vi "TextLog-Logging Thread.vi"(7 "length":i32=100000) -> ()   [LabVIEW 2020]
uses:
  TextLog-Queue Data.ctl
  TextLog-Command.ctl
  TextLog-State.ctl
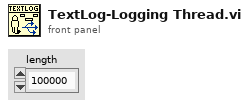
[diagram p1: front panel]
types:
  T1 = typedef "TextLog-State.ctl" = cluster{"path":path, "index":i32, "log":u8[], "length":i32, "logging":bool}
  T2 = typedef "TextLog-Queue Data.ctl" = cluster{"Time":string, "Command":T3, "Message":string, "Data":string}
  T3 = typedef "TextLog-Command.ctl" = enum16{"Unspecified", "Start", "Stop", "Quit", "Rename", "Make entry"}
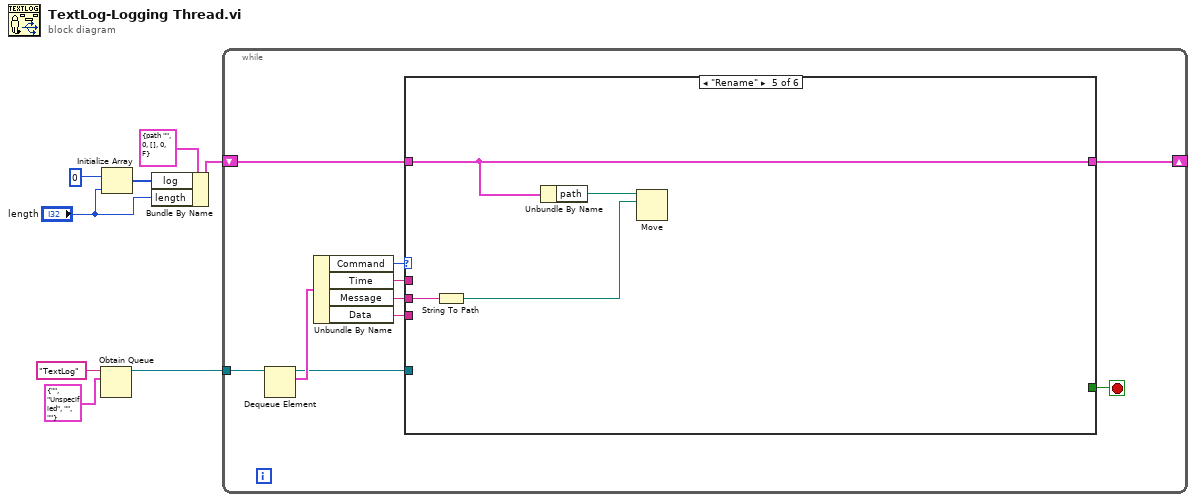
[diagram p0: block diagram]
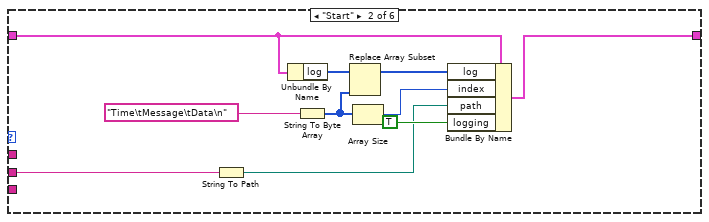
[diagram p3: hidden frame]
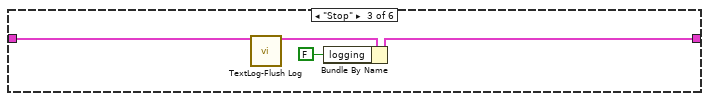
[diagram p4: hidden frame]
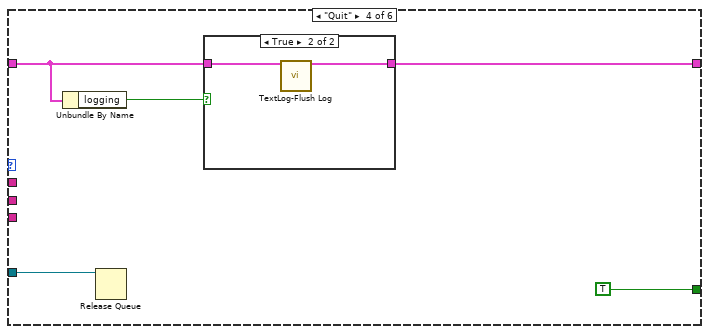
[diagram p5: hidden frame]
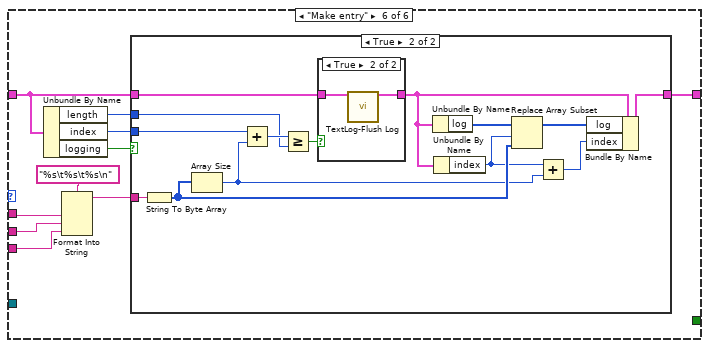
[diagram p7: hidden frame]
diagram:
  n1 = Obtain Queue(name (unnamed)="TextLog", element data type=T2 {"Time"="", "Command"=enum."Unspecified", "Message"="", "Data"=""} ("Trace Data")) -> (queue out=w6:refnum<queue>)  [unwired: 3 in, 2 out]
  n2 = Initialize Array(u8 0, "length") -> (w1:u8[])
  n3 = Bundle By Name(cluster=T1 {"path"=path "", "index"=0, "log"=[], "length"=0, "logging"=FALSE} ("State"), "log"=w1, "length"="length") -> (w4:T1)
  n4 = while {
    tunnel: w6 -> [w18]
    shift-right: [w9] -> _
    shift-left: w4 -> [w12]
    stop <- w10 stop-if-true
    n5 = Dequeue Element(queue=w18) -> (queue out=w11:refnum<queue>, element=w17:T2)  [unwired: 2 in, 2 out]
    n6 = Unbundle By Name(w17) -> ("Command"=w16:T3, "Time"=w15:string, "Message"=w14:string, "Data"=w13:string)
    n7 = case shown="\"Rename\"" w16 {
      tunnel: [_ _ _ TRUE _ _] -> w10
      tunnel: w15 -> [_ _ _ _ _ w54]
      tunnel: w14 -> [_ w20 _ _ w43 w53]
      tunnel: w13 -> [_ _ _ _ _ w52]
      tunnel: w12 -> [w19 w22 w33 w35 w45 w48]
      tunnel: w11 -> [_ _ _ w38 _ _]
      tunnel: [w19 w21 w31 w34 w45 w47] -> w9
      frame "Unspecified", Default {
      }
      frame "Start" {
        n8 = String To Path(string=w20) -> (path=w25:path)
        n9 = Unbundle By Name(w22) -> ("log"=w23:u8[])
        n10 = String To Byte Array(string="Time\tMessage\tData\n") -> (unsigned byte array=w26:u8[])
        n11 = Replace Array Subset(array=w23, new element=w26) -> (w24:u8[])  [unwired: 1 in]
        n12 = Array Size(array=w26) -> (size(s)=w27:i32)
        n13 = Bundle By Name(cluster=w22, "log"=w24, "index"=w27, "path"=w25, "logging"=TRUE) -> (w21:T1)
      }
      frame "Stop" {
        n14 = call "TextLog-Flush Log.vi"("State in"=w33) -> ("State out"=w32:T1)  [unwired: 14 in]
        n15 = Bundle By Name(cluster=w32, "logging"=FALSE) -> (w31:T1)
      }
      frame "Quit" {
        n16 = Unbundle By Name(w35) -> ("logging"=w36:bool)
        n17 = Release Queue(queue=w38) -> ()  [unwired: 2 in, 3 out]
        n18 = case shown="True" w36 {
          tunnel: w35 -> [w39 w41]
          tunnel: [w39 w40] -> w34
          frame False {
          }
          frame True {
            n19 = call "TextLog-Flush Log.vi"("State in"=w41) -> ("State out"=w40:T1)  [unwired: 14 in]
          }
        }
      }
      frame "Rename" {
        n20 = String To Path(string=w43) -> (path=w42:path)
        n21 = Unbundle By Name(w45) -> ("path"=w44:path)
        n22 = Move(source path=w44, 10:w42) -> ()  [unwired: 3 in, 3 out]
      }
      frame "Make entry" {
        n23 = Unbundle By Name(w48) -> ("length"=w49:i32, "index"=w50:i32, "logging"=w46:bool)
        n24 = Format Into String(format string="%s\t%s\t%s\n", w54, w53, w52) -> (resulting string=w51:string)  [unwired: 2 in, 1 out]
        n25 = case shown="True" w46 {
          tunnel: w51 -> [_ w70]
          tunnel: w50 -> [_ w69]
          tunnel: w49 -> [_ w67]
          tunnel: w48 -> [w56 w65]
          tunnel: [w56 w62] -> w47
          frame False {
          }
          frame True {
            n26 = String To Byte Array(string=w70) -> (unsigned byte array=w63:u8[])
            n27 = Array Size(array=w63) -> (size(s)=w57:i32)
            n28 = Add(x=w69, y=w57) -> (x+y=w68:i32)
            n29 = Greater Or Equal?(x=w68, y=w67) -> (x >= y?=w66:bool)
            n30 = case shown="True" w66 {
              tunnel: w65 -> [w71 w73]
              tunnel: [w71 w72] -> w60
              frame False {
              }
              frame True {
                n31 = call "TextLog-Flush Log.vi"("State in"=w73) -> ("State out"=w72:T1)  [unwired: 14 in]
              }
            }
            n32 = Unbundle By Name(w60) -> ("log"=w64:u8[])
            n33 = Unbundle By Name(w60) -> ("index"=w59:i32)
            n34 = Replace Array Subset(array=w64, new element=w63, index=w59) -> (w61:u8[])
            n35 = Add(x=w59, y=w57) -> (x+y=w58:i32)
            n36 = Bundle By Name(cluster=w60, "log"=w61, "index"=w58) -> (w62:T1)
          }
        }
      }
    }
  }
